vi "park mirrors.vi"() -> ()   [LabVIEW 2012]
doc: "SciScan 1.2 160622"
panel:
  in  "y mirror":dbl(slide) scale=-2.0..2.0
  in  "x mirror":dbl(slide) scale=-2.0..2.0
  in  "stop":bool
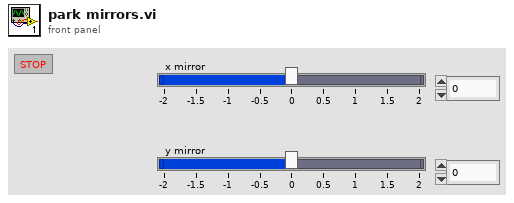
[diagram p1: front panel]
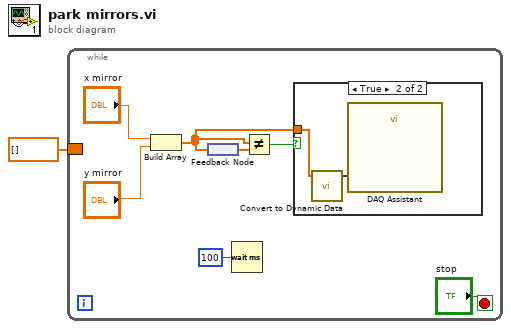
[diagram p0: block diagram]
diagram:
  n1 = while {
    border: dbl[] [] -> [_]
    stop <- "stop" stop-if-true
    n2 = Build Array("x mirror", "y mirror") -> (w2:dbl[])
    n3 = feedback-in #1(w2) -> ()
    n4 = feedback #1() -> (w4:dbl[])
    n5 = Wait (ms)(milliseconds to wait=u32 100) -> ()  [unwired: 1 out]
    n6 = Not Equal?(x=w2, y=w4) -> (x != y?=w5:bool)
    n7 = case shown="True" w5 {
      tunnel: w2 -> [_ w10]
      frame False {
      }
      frame True {
        n8 = call "Convert to Dynamic Data"("Array"=w10) -> ("Dynamic Data Type"=w9:dynamicdata)  [unwired: 3 in]
        n9 = call "DAQ Assistant"("data"=w9) -> ()  [unwired: 17 in, 2 out]
      }
    }
  }
